vi "Create or Add Phrase or Paragraph with Images.vi"(0 "Leading":sgl=12.0, 1 "Phrase or paragraph":T3, 2 "Text zone (points)":cluster{"widht":sgl, "height":sgl}={"widht"=612.0, "height"=792.0}, 3 "Character type":T1=enum."ASCII", 5 "Phrase refnum IN":refnum<k24>, 7 "Paragraph refnum IN":refnum<k24>, 9 "Text":string, 11 "error in (no error)":errorcluster, 12 "Font refnum":refnum<k24>, 13 "Paragraph indentation (points)":T4, 14 "Image to Add refnum [ ]":T2) -> (4 "Leading duplicate":sgl=12.0, 6 "Phrase refnum OUT":refnum<k24>, 8 "Paragraph refnum OUT":refnum<k24>, 10 "Image?":bool, 15 "error out":errorcluster)   [LabVIEW 2020, in "Exaprom PDF.lvlib"]
doc: "Version 2.0\nDeveloped by Jean-Marc Simard\nCopyright © 2012, Exaprom Inc.\nAll rights reserved.\nLicense: BSD\n\nWith iTextSharp 4.1.6 (http://itextsharp.sourceforge.net)\nunder Mozilla Public License Version 1.1\n(http://www.mozilla.org/MPL/MPL-1.1.html)"
uses:
  <userlib>/labview-PDF-writer-master/Exaprom PDF.lvlib
  C:/Program Files (x86)/National Instruments/LabVIEW 2020/user.lib/labview-PDF-writer-master/DLL/itextsharp.dll
  DLL/itextsharp.dll
  <userlib>/labview-PDF-writer-master/Controls/Text Controls/Paragraph indentation.ctl
  <userlib>/labview-PDF-writer-master/Controls/Text Controls/Phrase or paragraph.ctl
  <userlib>/labview-PDF-writer-master/Controls/General Controls/Image to Add refnum [ ].ctl
  <userlib>/labview-PDF-writer-master/Controls/Text Controls/Unicode/Type and run direction.ctl
  <userlib>/labview-PDF-writer-master/Controls/Image Controls/Image Scale Type.ctl
  <userlib>/labview-PDF-writer-master/LV Class/Fonts Class/Font Class.lvclass
panel:
  # "Add to Phrase  添加到短语\nAdd to Paragraph 增加一段\nCreate Phrase 创建的短语\nCreate Paragraph 创建段落"
  # "文本区(点)"
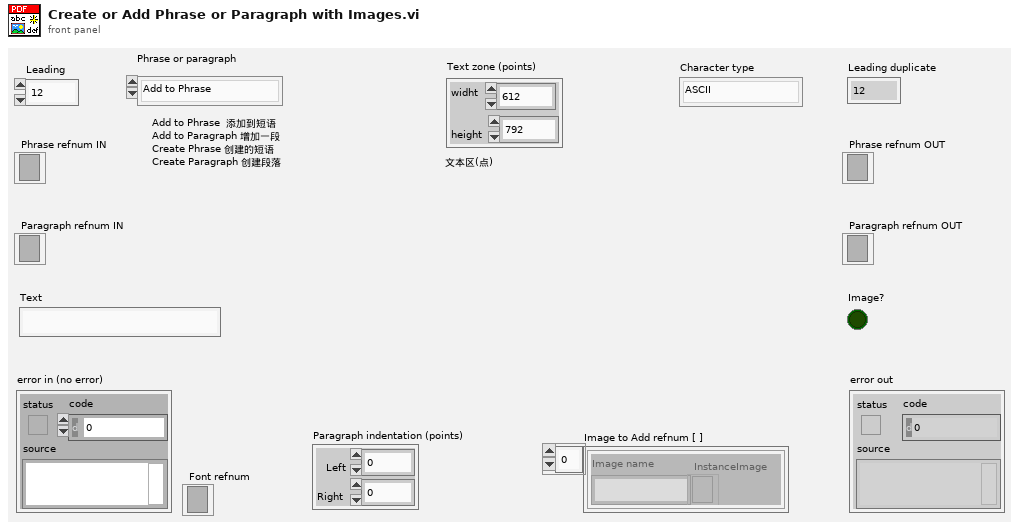
[diagram p1: front panel]
types:
  T1 = typedef "Exaprom PDF.lvlib/Type and run direction.ctl" = enum16{"Select", "ASCII", "UTF-16", "UTF-16 (default)", "UTF-16 (LTR)", "UTF-16 (RTL)"}
  T2 = typedef "Exaprom PDF.lvlib/Image to Add refnum [ ].ctl" = cluster{"Image name":string, "InstanceImage":refnum<k24>}[]
  T3 = typedef "Exaprom PDF.lvlib/Phrase or paragraph.ctl" = enum16{"Add to Phrase", "Add to Paragraph", "Create Phrase", "Create Paragraph"}
  T4 = typedef "Exaprom PDF.lvlib/Paragraph indentation.ctl" = cluster{"Left":sgl, "Right":sgl}
  T5 = typedef "Exaprom PDF.lvlib/Image Scale Type.ctl" = enum16{"%", "Height", "Width"}
  T6 = typedef "Exaprom PDF.lvlib/Text element type.ctl" = enum16{"Text", "Image", "Not a valid image", "Link"}
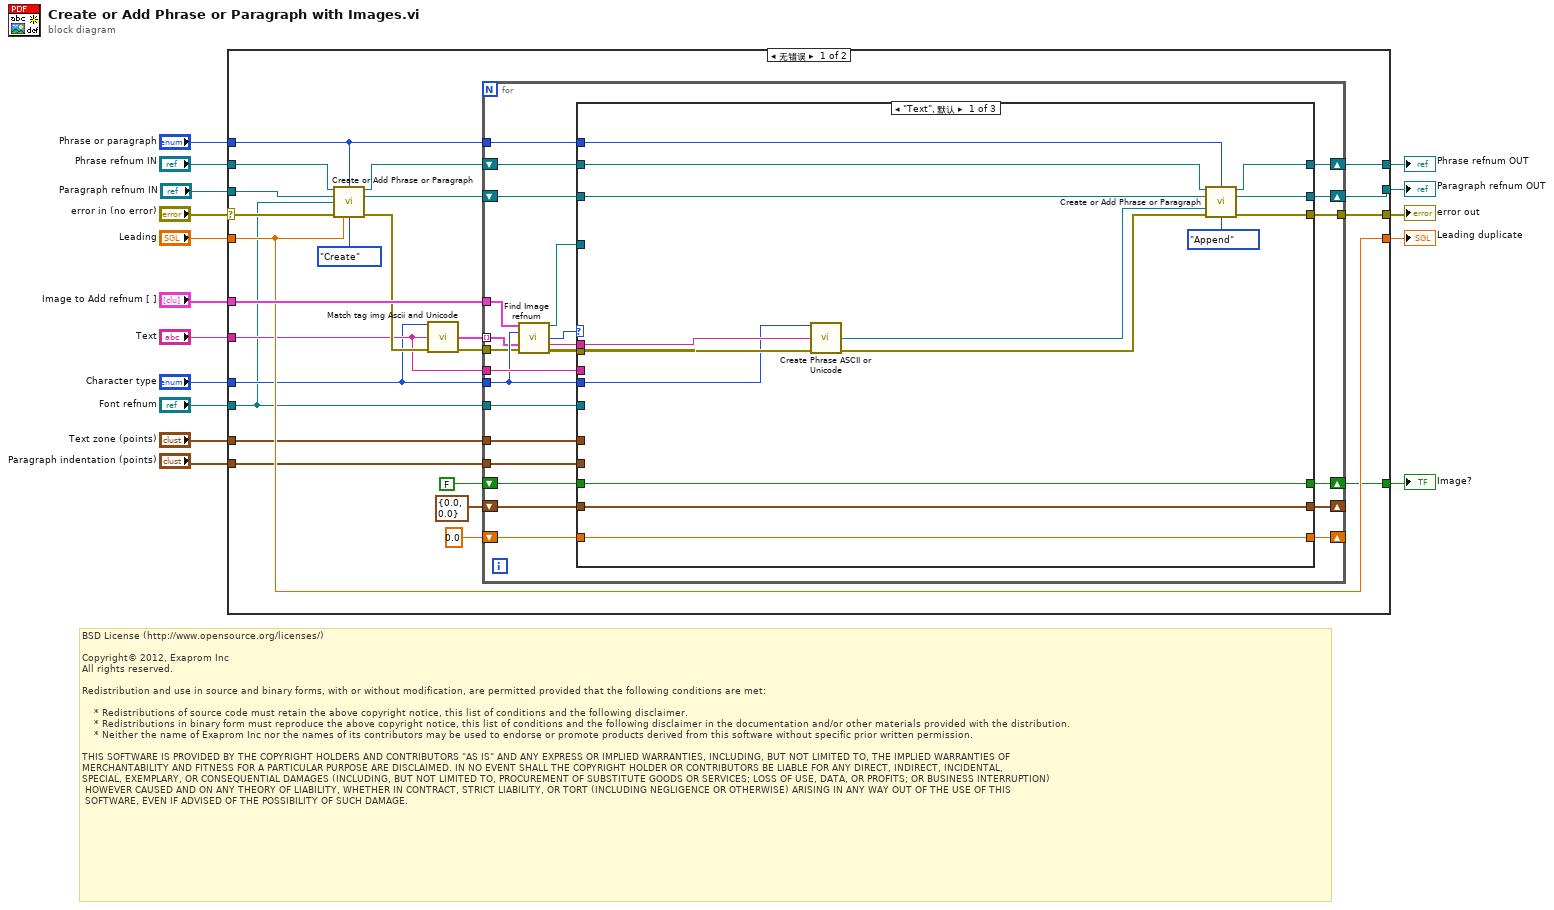
[diagram p0: block diagram]
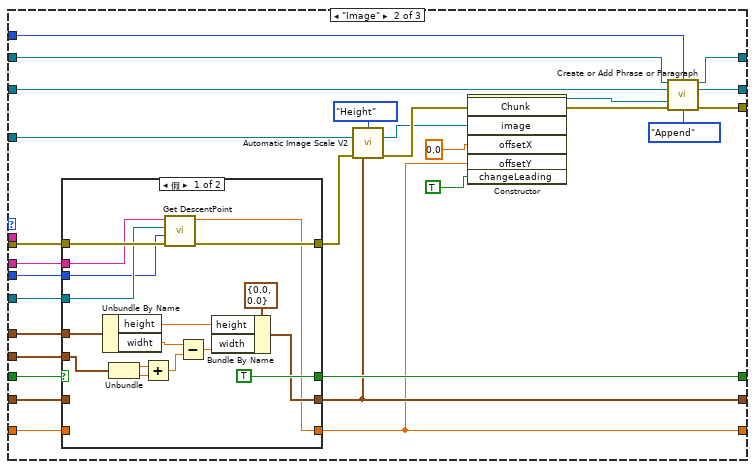
[diagram p2: hidden frame]
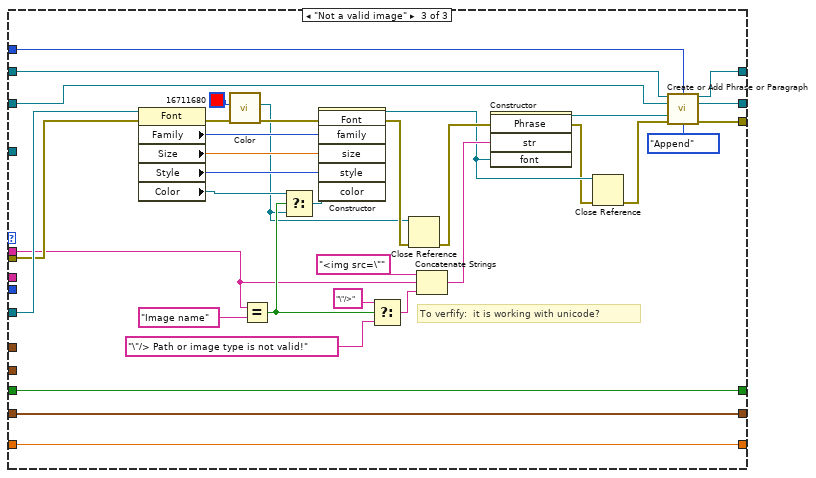
[diagram p4: hidden frame]
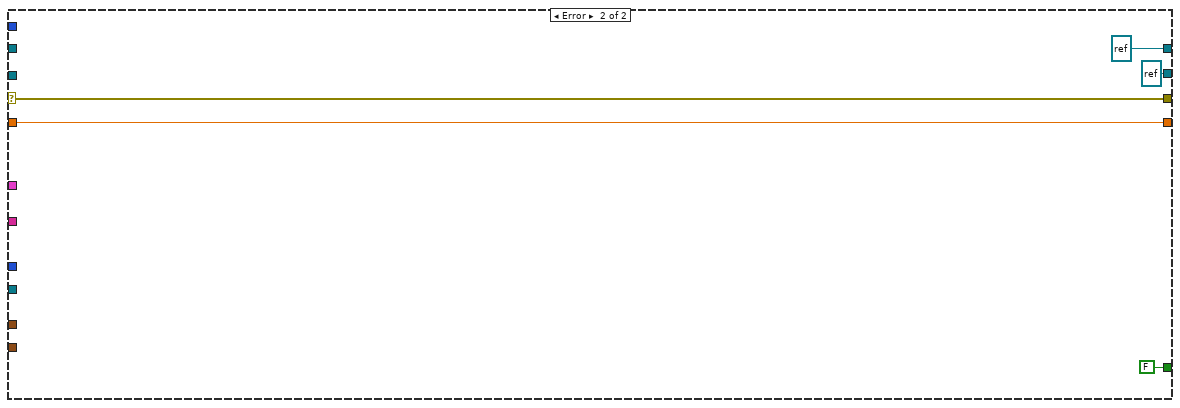
[diagram p5: hidden frame]
diagram:
  # "BSD License (http://www.opensource.org/licenses/)\n\nCopyright© 2012, Exaprom Inc\nAll rights reserved.\n\nRedistribution and use in source and binary forms, with or without modification, are permitted provided that the following conditions are met:\n\n    * Redistributions of source code must retain the above copyright notice, this list of conditions and the following disclaimer.\n    * Redistributions in binary form must reproduce the above copyright notice, this list of conditions and the following disclaimer in the documentation and/or other materials provided with the distribution.\n    * Neither the name of Exaprom Inc nor the names of its contributors may be used to endorse or promote products derived from this software without specific prior written permission.\n\nTHIS SOFTWARE IS PROVIDED BY THE COPYRIGHT HOLDERS AND CONTRIBUTORS \"AS IS\" AND ANY EXPRESS OR IMPLIED WARRANTIES, INCLUDING, BUT NOT LIMITED TO, THE IMPLIED WARRANTIES OF \nMERCHANTABILITY AND FITNESS FOR A PARTICULAR PURPOSE ARE DISCLAIMED. IN NO EVENT SHALL THE COPYRIGHT HOLDER OR CONTRIBUTORS BE LIABLE FOR ANY DIRECT, INDIRECT, INCIDENTAL,\nSPECIAL, EXEMPLARY, OR CONSEQUENTIAL DAMAGES (INCLUDING, BUT NOT LIMITED TO, PROCUREMENT OF SUBSTITUTE GOODS OR SERVICES; LOSS OF USE, DATA, OR PROFITS; OR BUSINESS INTERRUPTION)\n HOWEVER CAUSED AND ON ANY THEORY OF LIABILITY, WHETHER IN CONTRACT, STRICT LIABILITY, OR TORT (INCLUDING NEGLIGENCE OR OTHERWISE) ARISING IN ANY WAY OUT OF THE USE OF THIS\n SOFTWARE, EVEN IF ADVISED OF THE POSSIBILITY OF SUCH DAMAGE."
  n1 = case shown="无错误" "error in (no error)" {
    selector: "error in (no error)" -> [w35 w168]
    tunnel: "Image to Add refnum [ ]" -> [w40 _]
    tunnel: "Text" -> [w24 _]
    tunnel: [w33 refnum<k24> refnum ("new reference")] -> w6
    tunnel: "Leading" -> [w31 w165]
    tunnel: "Font refnum" -> [w20 _]
    tunnel: [w32 w168] -> w12
    tunnel: "Text zone (points)" -> [w25 _]
    tunnel: "Paragraph indentation (points)" -> [w26 _]
    tunnel: "Phrase or paragraph" -> [w18 _]
    tunnel: [w34 refnum<k24> refnum ("new reference")] -> w7
    tunnel: [w31 w165] -> w9
    tunnel: "Phrase refnum IN" -> [w28 _]
    tunnel: "Paragraph refnum IN" -> [w27 _]
    tunnel: [w22 FALSE] -> w3
    tunnel: "Character type" -> [w21 _]
    frame No Error {
      n2 = call <userlib>:"Create or Add Phrase or Paragraph.vi"("Phrase refnum IN"=w28, "Phrase or paragraph"=w18, "Paragraph refnum IN"=w27, "Font refnum"=w20, "error in (no error)"=w35, "Leading"=w31, "Only"=enum16{"Create", "Append"}."Create") -> ("Phrase refnum OUT"=w36:refnum<k24>, "Paragraph refnum OUT"=w38:refnum<k24>, "error out"=w37:errorcluster)  [unwired: 6 in]
      n3 = call <userlib>:"Match tag img Ascii and Unicode.vi"("Type and run direction"=w21, "String"=w24, "error in (no error)"=w37) -> ("Text [ ]"=w17:cluster{"ASCII":string, "Image?":bool}[], "error out"=w39:errorcluster)  [unwired: 11 in]
      n4 = for {
        tunnel: w17 -> [w41] mode=indexing
        shift-right: [w51] -> w33
        shift-left: w38 -> [w64]
        tunnel: w40 -> [w48]
        tunnel: w39 -> [w46]
        tunnel: [w50] -> w32
        tunnel: w26 -> [w63]
        shift-right: [w52] -> w34
        shift-left: w36 -> [w62]
        tunnel: w18 -> [w49]
        tunnel: w20 -> [w61]
        shift-right: [w57] -> w22
        shift-left: FALSE -> [w58]
        shift-right: [w54] -> _
        shift-left: sgl 0.0 ("GetDescentPoint") -> [w53]
        tunnel: w25 -> [w60]
        tunnel: w24 -> [w59]
        shift-right: [w56] -> _
        shift-left: cluster{"width":sgl, "height":sgl} {"width"=0.0, "height"=0.0} ("Box") -> [w55]
        tunnel: w21 -> [w47]
        n5 = call <userlib>:"Find Image refnum.vi"("Image to Add refnum [ ]"=w48, "Type and run direction"=w47, "Text cluster"=w41, "error in (no error)"=w46) -> ("InstanceImage refnum"=w43:refnum<k24>, "Text element type"=w44:T6, "Text Duplicate"=w42:string, "error out"=w45:errorcluster)  [unwired: 7 in, 1 out]
        n6 = case shown="\"Text\", 默认" w44 {
          tunnel: [w71 w93 w138] -> w51
          tunnel: w64 -> [w75 w91 w132]
          tunnel: w45 -> [w69 w103 w155]
          tunnel: [w76 w94 w139] -> w50
          tunnel: w63 -> [_ w105 _]
          tunnel: w49 -> [w73 w89 w134]
          tunnel: w62 -> [w74 w90 w135]
          tunnel: [w72 w92 w137] -> w52
          tunnel: w61 -> [_ w102 w159]
          tunnel: w43 -> [_ w84 _]
          tunnel: w60 -> [_ w104 _]
          tunnel: w59 -> [_ w101 _]
          tunnel: w58 -> [w79 w100 w142]
          tunnel: [w79 w99 w142] -> w57
          tunnel: [w78 w97 w141] -> w56
          tunnel: w55 -> [w78 w98 w141]
          tunnel: [w77 w95 w140] -> w54
          tunnel: w53 -> [w77 w96 w140]
          tunnel: w47 -> [w65 w80 _]
          tunnel: w42 -> [w66 _ w129]
          frame "Text", Default {
            n7 = call <userlib>:"Create Phrase ASCII or Unicode.vi"("Character type"=w65, "Text"=w66, "error in (no error)"=w69) -> ("Phrase refnum"=w67:refnum<k24>, "error out"=w68:errorcluster)  [unwired: 10 in, 1 out]
            n8 = call <userlib>:"Create or Add Phrase or Paragraph.vi"("Phrase refnum IN"=w74, "Phrase or paragraph"=w73, "Paragraph refnum IN"=w75, "value"=w67, "error in (no error)"=w68, "Only"=enum16{"Create", "Append"}."Append") -> ("Phrase refnum OUT"=w72:refnum<k24>, "Paragraph refnum OUT"=w71:refnum<k24>, "error out"=w76:errorcluster)  [unwired: 7 in]
          }
          frame "Image" {
            n9 = case shown="假" w100 {
              selector: w100 -> [_ w127]
              tunnel: w105 -> [w119 _]
              tunnel: w104 -> [w118 _]
              tunnel: [w117 w128] -> w85
              tunnel: w103 -> [w116 w128]
              tunnel: w102 -> [w115 _]
              tunnel: w101 -> [w114 _]
              tunnel: [TRUE w127] -> w99
              tunnel: [w112 w126] -> w97
              tunnel: w98 -> [_ w126]
              tunnel: [w111 w125] -> w95
              tunnel: w96 -> [_ w125]
              tunnel: w80 -> [w108 _]
              frame False {
                n10 = Unbundle By Name(w118) -> ("height"=w110:sgl, "widht"=w109:sgl)
                n11 = Unbundle(w119) -> ("Left"=w124:sgl, "Right"=w123:sgl)
                n12 = Add(x=w124, y=w123) -> (x+y=w122:sgl)
                n13 = call <userlib>:"Get DescentPoint.vi"("error in (no error)"=w116, "Character type"=w108, "Font refnum"=w115, "String"=w114) -> ("error out"=w117:errorcluster, "DescentPoint"=w111:sgl)  [unwired: 6 in]
                n14 = Subtract(x=w109, y=w122) -> (x-y=w121:sgl)
                n15 = Bundle By Name(cluster=cluster{"width":sgl, "height":sgl} {"width"=0.0, "height"=0.0} ("Box"), "height"=w110, "width"=w121) -> (w112:cluster{"width":sgl, "height":sgl})
              }
              frame True {
              }
            }
            n16 = call <userlib>:"Automatic Image Scale V2.vi"("Scale Type"=Image_Scale_Type."Height", "GetInstanceImage IN"=w84, "error in (no error)"=w85, "Box"=w97) -> ("GetInstanceImage OUT"=w83:refnum<k24>, "error out"=w86:errorcluster)  [unwired: 7 in, 3 out]
            n17 = constructor class="Chunk"(error in=w86, "image"=w83, "offsetX"=sgl 0.0, "offsetY"=w95, "changeLeading"=TRUE) -> (reference out=w88:refnum<k24>, error out=w81:errorcluster)  [unwired: 2 in, 5 out]
            n18 = call <userlib>:"Create or Add Phrase or Paragraph.vi"("Phrase refnum IN"=w90, "Phrase or paragraph"=w89, "Paragraph refnum IN"=w91, "value"=w88, "error in (no error)"=w81, "Only"=enum16{"Create", "Append"}."Append") -> ("Phrase refnum OUT"=w92:refnum<k24>, "Paragraph refnum OUT"=w93:refnum<k24>, "error out"=w94:errorcluster)  [unwired: 7 in]
          }
          frame "Not a valid image" {
            # "To verfify:  it is working with unicode?"
            n19 = property class="Font"(reference=w159, error in=w155) -> (error out=w158:errorcluster, "Family"=w153:i32, "Size"=w152:sgl, "Style"=w151:i32, "Color"=w144:refnum<k24>)  [unwired: 1 out]
            n20 = call <userlib>:"Color.vi"("error in (no error)"=w158, "Color"=u32 16711680) -> ("error out"=w154:errorcluster, "Color"=w143:refnum<k24>)  [unwired: 8 out]
            n21 = Equal?(x=w129, y="Image name" ("x")) -> (x = y?=w145:bool)
            n22 = Select(t=w144, s=w145, f=w143) -> (s? t:f=w146:refnum<k24>)
            n23 = constructor class="Font"(error in=w154, "family"=w153, "size"=w152, "style"=w151, "color"=w146) -> (reference out=w148:refnum<k24>, error out=w150:errorcluster)  [unwired: 2 in, 5 out]
            n24 = Select(t="\"/>", s=w145, f="\"/> Path or image type is not valid!") -> (s? t:f=w162:string)
            n25 = Close Reference(reference=w143, error in (no error)=w150) -> (error out=w149:errorcluster)
            n26 = Concatenate Strings("<img src=\"", w129, w162) -> (w156:string)
            n27 = constructor class="Phrase"(error in=w149, "str"=w156, "font"=w148) -> (reference out=w133:refnum<k24>, error out=w147:errorcluster)  [unwired: 2 in, 3 out]
            n28 = Close Reference(reference=w148, error in (no error)=w147) -> (error out=w136:errorcluster)
            n29 = call <userlib>:"Create or Add Phrase or Paragraph.vi"("Phrase refnum IN"=w135, "Phrase or paragraph"=w134, "Paragraph refnum IN"=w132, "value"=w133, "error in (no error)"=w136, "Only"=enum16{"Create", "Append"}."Append") -> ("Phrase refnum OUT"=w137:refnum<k24>, "Paragraph refnum OUT"=w138:refnum<k24>, "error out"=w139:errorcluster)  [unwired: 7 in]
          }
        }
      }
    }
    frame Error {
    }
  }
  "error out" <- w12
  "Paragraph refnum OUT" <- w6
  "Phrase refnum OUT" <- w7
  "Leading duplicate" <- w9
  "Image?" <- w3
